vi "Word_Insert_Footer.vi"(0 "Word._Document":refnum<k7>, 1 "font":T1 {"font size" format="%.2f"; "strike through" items=["Strk Unchanged", "Strk Yes", "Strk No"]; "underline" items=["Und Unchanged", "Und Yes", "Und No"]; "italic" items=["Ital Unchanged", "Ital Yes", "Ital No"]; "bold" items=["Bold Unchanged", "Bold Yes", "Bold No"]}, 5 "Left text":string, 7 "Central text":string, 9 "Right text":string, 11 "Error In (no error)":errorcluster) -> (15 "Error Out":errorcluster)   [LabVIEW 2020, in "NI_ReportGenerationToolkit.lvlib"]
uses:
  <vilib>/addons/_office/NI_ReportGenerationToolkit.lvlib
  <vilib>/addons/_office/_exclsub.llb/font.ctl
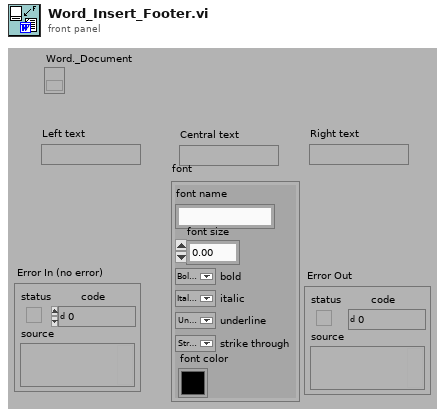
[diagram p1: front panel]
types:
  T1 = typedef "NI_ReportGenerationToolkit.lvlib/font.ctl" = cluster{"font name":string, "font size":dbl, "bold":u16, "italic":u16, "underline":u16, "strike through":u16, "font color":u32}
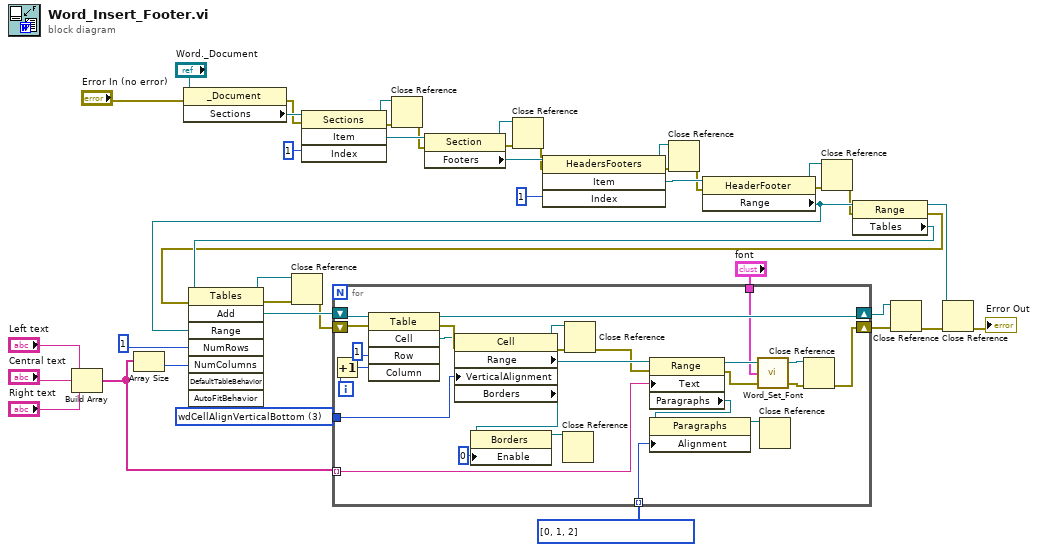
[diagram p0: block diagram]
diagram:
  w12 = 3 items=["wdCellAlignVerticalTop"=0, "wdCellAlignVerticalCenter"=1, "wdCellAlignVerticalBottom"=3] ("VerticalAlignment")
  w11 = i32[] [0, 1, 2] items=["wdAlignParagraphLeft"=0, "wdAlignParagraphCenter"=1, "wdAlignParagraphRight"=2, "wdAlignParagraphJustify"=3, "wdAlignParagraphDistribute"=4, "wdAlignParagraphJustifyMed"=5, "wdAlignParagraphJustifyHi"=7, "wdAlignParagraphJustifyLow"=8] ("Array Constant")
  n1 = Build Array("Left text", "Central text", "Right text") -> (w29:string[])
  n2 = Array Size(array=w29) -> (size(s)=w34:i32)
  n3 = property class="_Document"(reference="Word._Document", error in="Error In (no error)") -> (error out=w21:errorcluster, "Sections"=w42:refnum<k7>)  [unwired: 1 out]
  n4 = invoke class="Sections" method="Item"(reference=w42, error in=w21, "Index"=1) -> (reference out=w27:refnum<k7>, error out=w28:errorcluster, "Item"=w41:refnum<k7>)  [unwired: 1 in, 1 out]
  n5 = Close Reference(reference=w27, error in (no error)=w28) -> (error out=w26:errorcluster)
  n6 = property class="Section"(reference=w41, error in=w26) -> (reference out=w24:refnum<k7>, error out=w25:errorcluster, "Footers"=w37:refnum<k7>)
  n7 = Close Reference(reference=w24, error in (no error)=w25) -> (error out=w23:errorcluster)
  n8 = invoke class="HeadersFooters" method="Item"(reference=w37, error in=w23, "Index"=1) -> (reference out=w19:refnum<k7>, error out=w20:errorcluster, "Item"=w39:refnum<k7>)  [unwired: 1 in, 1 out]
  n9 = Close Reference(reference=w19, error in (no error)=w20) -> (error out=w18:errorcluster)
  n10 = property class="HeaderFooter"(reference=w39, error in=w18) -> (reference out=w16:refnum<k7>, error out=w17:errorcluster, "Range"=w36:refnum<k7>)
  n11 = Close Reference(reference=w16, error in (no error)=w17) -> (error out=w15:errorcluster)
  n12 = property class="Range"(reference=w36, error in=w15) -> (reference out=w3:refnum<k7>, error out=w6:errorcluster, "Tables"=w33:refnum<k7>)
  n13 = invoke class="Tables" method="Add"(reference=w33, error in=w6, "Range"=w36, "NumRows"=1, "NumColumns"=w34) -> (reference out=w13:refnum<k7>, error out=w14:errorcluster, "Add"=w10:refnum<k7>)  [unwired: 3 in, 5 out]
  n14 = Close Reference(reference=w13, error in (no error)=w14) -> (error out=w7:errorcluster)
  n15 = for {
    shift-right: [w45] -> w8
    shift-left: w7 -> [w53]
    tunnel: w29 -> [w65] mode=indexing
    tunnel: w12 -> [w58]
    tunnel: w11 -> [w57] mode=indexing
    shift-right: [w54] -> w9
    shift-left: w10 -> [w55]
    tunnel: "font" -> [w43]
    i -> [w68]
    n16 = Increment(x=w68) -> (x+1=w67:i32)
    n17 = invoke class="Table" method="Cell"(reference=w55, error in=w53, "Row"=1, "Column"=w67) -> (reference out=w54:refnum<k7>, error out=w62:errorcluster, "Cell"=w61:refnum<k7>)  [unwired: 1 in, 2 out]
    n18 = property class="Cell"(reference=w61, error in=w62, "VerticalAlignment"=w58) -> (reference out=w51:refnum<k7>, error out=w52:errorcluster, "Range"=w50:refnum<k7>, "Borders"=w60:refnum<k7>)
    n19 = property class="Borders"(reference=w60, "Enable"=0) -> (reference out=w48:refnum<k7>)  [unwired: 1 in, 1 out]
    n20 = Close Reference(reference=w48) -> ()  [unwired: 1 in, 1 out]
    n21 = Close Reference(reference=w51, error in (no error)=w52) -> (error out=w49:errorcluster)
    n22 = property class="Range"(reference=w50, error in=w49, "Text"=w65) -> (reference out=w64:refnum<k7>, error out=w63:errorcluster, "Paragraphs"=w56:refnum<k7>)
    n23 = property class="Paragraphs"(reference=w56, "Alignment"=w57) -> (reference out=w47:refnum<k7>)  [unwired: 1 in, 1 out]
    n24 = call <vilib>:"Word_Set_Font.vi"("Range in"=w64, "font"=w43, "Error in"=w63) -> ("Range out"=w44:refnum<k7>, "Error out"=w46:errorcluster)  [unwired: 5 out]
    n25 = Close Reference(reference=w47) -> ()  [unwired: 1 in, 1 out]
    n26 = Close Reference(reference=w44, error in (no error)=w46) -> (error out=w45:errorcluster)
  }
  n27 = Close Reference(reference=w9, error in (no error)=w8) -> (error out=w5:errorcluster)
  n28 = Close Reference(reference=w3, error in (no error)=w5) -> (error out=→"Error Out":errorcluster)
